vi "Power - Continuous Measurement.vi"() -> ()   [LabVIEW 2022 SP3]
doc: "This example demonstrates how to continuously acquire buffered power measurements using a DAQmx device.\n\nFor instructions on how to connect your signals to the DAQ device, refer to your device documentation."
uses:
  <vilib>/Utility/error.llb/DialogType.ctl
  <vilib>/DAQmx/read.llb/DAQmx Read (Power 2D DBL NChan NSamp).vi
  <vilib>/DAQmx/create/channels.llb/DAQmx Create Channel (Power).vi
  <vilib>/DAQmx/configure/timing.llb/DAQmx Timing (Sample Clock).vi
  <vilib>/DAQmx/configure/trigger.llb/DAQmx Start Trigger (Digital Edge).vi
  <vilib>/DAQmx/miscellaneous.llb/DAQmx Fill In Error Info.vi
  <resource>/objmgr/daqmx.rc
panel:
  in  "Physical Channel":tag="TS1Mod1/power"
  out "Overtemperature Channels":string[](array[string])
  out "Overtemperature Channels Exist":bool
  out "Output State":i32(ring)=15503 items=["Constant Voltage"=15500, "Constant Current"=15501, "Overvoltage"=15502, "Output Disabled"=15503]
  in  "Remote Sense":i32(ring)=16095 items=["Local"=16095, "Remote"=16096]
  in  "Idle Output Behavior":i32(ring)=15503 items=["Output Disabled"=15503, "Maintain Existing Value"=12528]
  in  "Update":bool
  in  "Output Enable":bool=TRUE
  in  "Voltage Setpoint":dbl=6.0
  in  "Current Setpoint":dbl=3.0
  in  "Stop":bool
  in  "Initial Output Enable":bool=TRUE
  in  "Trigger Type":T1(tab)
  in  "Digital Start Trigger Edge":i32(ring)=10280 caption="Edge" items=["Rising"=10280, "Falling"=10171]
  in  "Digital Start Trigger Source":tag="/TS1Mod2/PFI0" caption="Source"
  in  "Digital Pause Trigger Pause When":i32(ring)=10192 caption="Pause When" items=["High"=10192, "Low"=10214]
  in  "Digital Pause Trigger Source":tag="/TS1Mod2/PFI0" caption="Source"
  in  "Number of Samples":i32=100
  in  "Sample Rate":dbl=1000.0
  in  "Sample Clock Source":tag="OnboardClock"
  in  "Initial Voltage Setpoint":dbl=6.0
  in  "Initial Current Setpoint":dbl=3.0
  out "Actual Sample Rate":dbl=1000.0 format="%0.2f"
  out "Voltage Waveform Graph":dbl[][](graph)
  out "Current Waveform Graph":dbl[][](graph)
  # "Channel Settings"
  # "Acquired Voltage Data"
  # "Acquired Current Data"
  # "Timing Settings"
  # "Status"
  # "Trigger Settings"
  # "Runtime Settings"
  # "To change the power configuration at runtime, change the control values above and then press Update, below."
  # "To enable triggers, select a tab above, and configure the settings.\n\nNot all hardware supports all trigger types. Refer to your device documentation for more information."
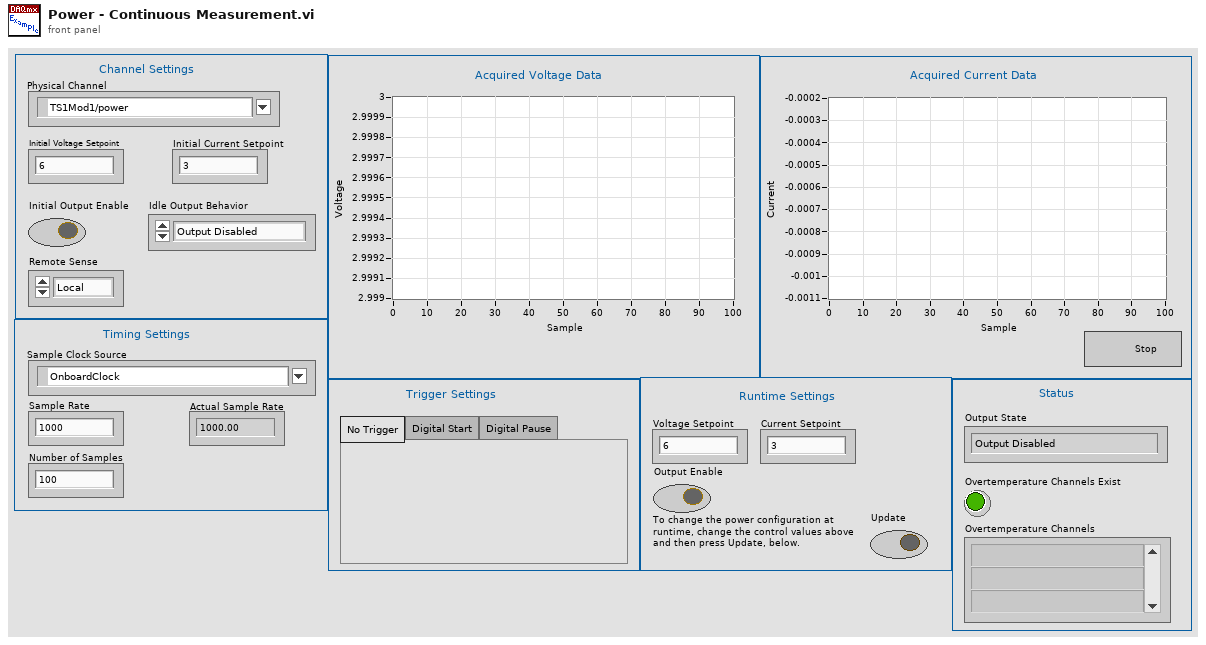
[diagram p1: front panel]
types:
  T1 = enum32{"No Trigger", "Digital Start", "Digital Pause"}
  T2 = typedef "DialogType.ctl" = u16
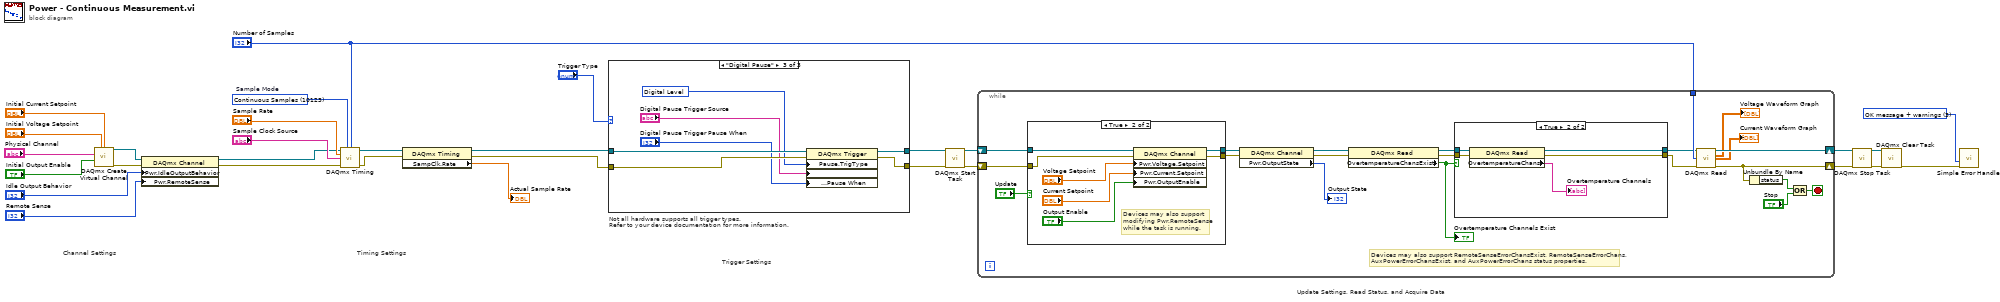
[diagram p0: block diagram]
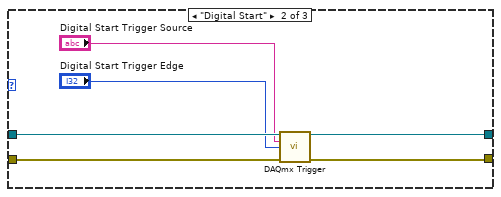
[diagram p5: hidden frame]
diagram:
  w13 = T2 3 items=["no dialog", "OK message", "continue or stop message", "OK message + warnings", "continue/stop + warnings"] ("type of dialog (OK msg:1)")
  w28 = 10123 items=["Finite Samples"=10178, "Continuous Samples"=10123, "Hardware Timed Single Point"=12522]  # Sample Mode
  # "Not all hardware supports all trigger types.\nRefer to your device documentation for more information."
  # "Trigger Settings"
  # "Update Settings, Read Status, and Acquire Data"
  # "Timing Settings"
  # "Channel Settings"
  n1 = call-poly <vilib>:"DAQmx Create Virtual Channel.vi"("voltage setpoint"="Initial Voltage Setpoint", "current setpoint"="Initial Current Setpoint", "physical channels"="Physical Channel", "output enable"="Initial Output Enable") -> ("task out"=w6:refnum<k21>, "error out"=w7:errorcluster)  [unwired: 10 in]
  n2 = property class="DAQmx Channel"(reference=w6, error in=w7, "Pwr.IdleOutputBehavior"="Idle Output Behavior", "Pwr.RemoteSense"="Remote Sense") -> (reference out=w3:refnum<k21>, error out=w4:errorcluster)
  n3 = call-poly <vilib>:"DAQmx Timing.vi"("task/channels in"=w3, "sample mode"=w28, "samples per channel"="Number of Samples", "rate"="Sample Rate", "source"="Sample Clock Source", "error in"=w4) -> ("task out"=w30:refnum<k21>, "error out"=w29:errorcluster)  [unwired: 8 in]
  n4 = property class="DAQmx Timing"(reference=w30, error in=w29) -> (reference out=w27:refnum<k21>, error out=w26:errorcluster, "SampClk.Rate"=→"Actual Sample Rate":dbl)
  n5 = case shown="\"Digital Pause\"" "Trigger Type" {
    tunnel: w27 -> [w32 w38 w45]
    tunnel: w26 -> [w31 w37 w42]
    tunnel: [w32 w36 w44] -> w11
    tunnel: [w31 w35 w43] -> w10
    frame "No Trigger", Default {
    }
    frame "Digital Start" {
      n6 = call-poly <vilib>:"DAQmx Trigger.vi"("task/channels in"=w38, "source"="Digital Start Trigger Source", "edge"="Digital Start Trigger Edge", "error in"=w37) -> ("task out"=w36:refnum<k21>, "error out"=w35:errorcluster)  [unwired: 10 in]
    }
    frame "Digital Pause" {
      w41 = 10152 items=["Analog Level"=10101, "Analog Window"=10103, "Digital Level"=10152, "Digital Pattern"=10398, "None"=10230] ("Pause.TrigType")
      n7 = property class="DAQmx Trigger"(reference=w45, error in=w42, "Pause.TrigType"=w41, "More:Pause:Digital Level:Source"="Digital Pause Trigger Source", "More:Pause:Digital Level:Pause When"="Digital Pause Trigger Pause When") -> (reference out=w44:refnum<k21>, error out=w43:errorcluster)
    }
  }
  n8 = call <vilib>:"DAQmx Start Task.vi"("task/channels in"=w11, "error in"=w10) -> ("task out"=w25:refnum<k21>, "error out"=w24:errorcluster)  [unwired: 12 in]
  n9 = while {
    shift-right: [w66] -> w15
    shift-left: w25 -> [w58]
    shift-right: [w63] -> w14
    shift-left: w24 -> [w59]
    tunnel: "Number of Samples" -> [w61]
    stop <- w65 stop-if-true
    # "Devices may also support RemoteSenseErrorChansExist, RemoteSenseErrorChans,\nAuxPowerErrorChansExist, and AuxPowerErrorChans status properties."
    n10 = case shown="True" "Update" {
      tunnel: w59 -> [w74 w82]
      tunnel: w58 -> [w75 w81]
      tunnel: [w75 w76] -> w57
      tunnel: [w74 w77] -> w56
      frame False {
      }
      frame True {
        # "Devices may also support\nmodifying Pwr.RemoteSense\nwhile the task is running."
        n11 = property class="DAQmx Channel"(reference=w81, error in=w82, "Pwr.Voltage.Setpoint"="Voltage Setpoint", "Pwr.Current.Setpoint"="Current Setpoint", "Pwr.OutputEnable"="Output Enable") -> (reference out=w76:refnum<k21>, error out=w77:errorcluster)
      }
    }
    n12 = property class="DAQmx Channel"(reference=w57, error in=w56) -> (reference out=w54:refnum<k21>, error out=w53:errorcluster, "Pwr.OutputState"=→"Output State":i32)
    n13 = property class="DAQmx Read"(reference=w54, error in=w53) -> (reference out=w51:refnum<k21>, error out=w52:errorcluster, "OvertemperatureChansExist"=w48:bool)
    "Overtemperature Channels Exist" <- w48
    n14 = case shown="True" w48 {
      tunnel: w52 -> [w67 w72]
      tunnel: w51 -> [w68 w73]
      tunnel: [w67 w70] -> w50
      tunnel: [w68 w69] -> w49
      frame False {
      }
      frame True {
        n15 = property class="DAQmx Read"(reference=w73, error in=w72) -> (reference out=w69:refnum<k21>, error out=w70:errorcluster, "OvertemperatureChans"=→"Overtemperature Channels":string[])
      }
    }
    n16 = call-poly <vilib>:"DAQmx Read.vi"("task/channels in"=w49, "number of samples per channel"=w61, "error in"=w50) -> ("task out"=w66:refnum<k21>, "voltage"=→"Voltage Waveform Graph":dbl[][], "current"=→"Current Waveform Graph":dbl[][], "error out"=w63:errorcluster)  [unwired: 9 in]
    n17 = Unbundle By Name(w63) -> ("status"=w62:bool)
    n18 = Or(x=w62, y="Stop") -> (x .or. y?=w65:bool)
  }
  n19 = call <vilib>:"DAQmx Stop Task.vi"("task/channels in"=w15, "error in"=w14) -> ("task out"=w17:refnum<k21>, "error out"=w16:errorcluster)  [unwired: 12 in]
  n20 = call <vilib>:"DAQmx Clear Task.vi"("task in"=w17, "error in"=w16) -> ("error out"=w23:errorcluster)  [unwired: 13 in]
  n21 = call <vilib>:"Simple Error Handler.vi"("type of dialog (OK msg:1)"=w13, "error in (no error)"=w23) -> ()  [unwired: 3 in, 5 out]
